vi "Read_Measures_STD.vi"(11 "file path (dialog if empty)":path) -> (0 "Settings and measures":T1 {"Measure_Array"."Measure_values" format="%#_5p"; "Measure_Array"."Setting_values" format="%#_5p"}, 3 "new file path":path)   [LabVIEW 2009]
uses:
  <vilib>/Utility/file.llb/Read From Spreadsheet File (DBL).vi
  <vilib>/Utility/file.llb/Read From Spreadsheet File (string).vi
  <vilib>/Utility/file.llb/Read From Spreadsheet File (I64).vi
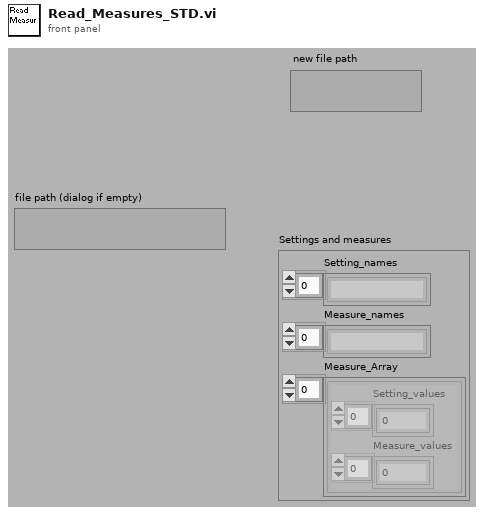
[diagram p1: front panel]
types:
  T1 = cluster{"Setting_names":string[], "Measure_names":string[], "Measure_Array":cluster{"Setting_values":dbl[], "Measure_values":dbl[]}[]}
  T2 = cluster{"Setting_values":dbl[], "Measure_values":dbl[]}
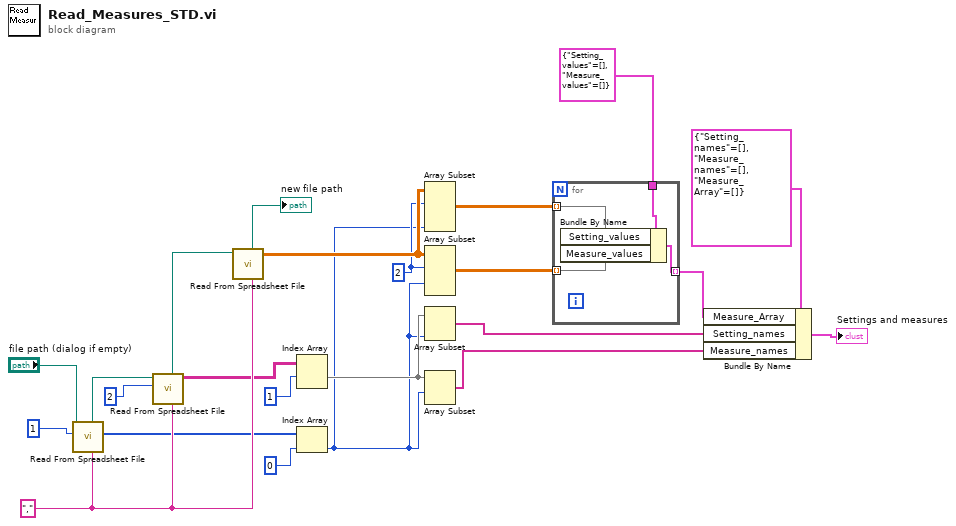
[diagram p0: block diagram]
diagram:
  w15 = 2 ("index")
  w20 = "," ("delimiter (\\t)")
  n1 = call-poly <vilib>:"Read From Spreadsheet File.vi"("delimiter (\\t)"=w20, "number of rows (all:-1)"=1, "file path (dialog if empty)"="file path (dialog if empty)") -> ("first row"=w18:i64[], "new file path (Not A Path if cancelled)"=w21:path)  [unwired: 4 in, 3 out]
  n2 = call-poly <vilib>:"Read From Spreadsheet File.vi"("delimiter (\\t)"=w20, "number of rows (all:-1)"=2, "file path (dialog if empty)"=w21) -> ("all rows"=w14:string[][], "new file path (Not A Path if cancelled)"=w23:path)  [unwired: 4 in, 3 out]
  n3 = call-poly <vilib>:"Read From Spreadsheet File.vi"("delimiter (\\t)"=w20, "file path (dialog if empty)"=w23) -> ("all rows"=w16:dbl[][], "new file path (Not A Path if cancelled)"=→"new file path":path)  [unwired: 5 in, 3 out]
  n4 = Index Array(array=w14, index (row)=1 ("index")) -> (element=w13:string[])  [unwired: 1 in]
  n5 = Index Array(array=w18, index=0) -> (element=w11:i64)
  n6 = Array Subset(array=w16, index (row)=w15, length (col)=w11) -> (w7:dbl[][])  [unwired: 2 in]
  n7 = Array Subset(array=w16, index (row)=w15, index (col)=w11) -> (w6:dbl[][])  [unwired: 2 in]
  n8 = Array Subset(array=w13, length=w11) -> (w8:string[])  [unwired: 1 in]
  n9 = Array Subset(array=w13, index=w11) -> (w9:string[])  [unwired: 1 in]
  n10 = for {
    tunnel: w7 -> [w26] mode=indexing
    tunnel: w6 -> [w25] mode=indexing
    tunnel: T2 {"Setting_values"=[], "Measure_values"=[]} ("Cluster") -> [w27]
    tunnel: [w24] -> w3 mode=indexing
    n11 = Bundle By Name(cluster=w27, "Setting_values"=w26, "Measure_values"=w25) -> (w24:T2)
  }
  n12 = Bundle By Name(cluster=T1 {"Setting_names"=[], "Measure_names"=[], "Measure_Array"=[]} ("Cluster 3"), "Measure_Array"=w3, "Setting_names"=w8, "Measure_names"=w9) -> (→"Settings and measures":T1)
